vi "7p1_HW_Task1B_doanbs.vi"(6 "Units":string, 9 "Convert?":string, 10 "th, Theta":dbl, 11 "Trig Function":string) -> (2 "Calculated Value":dbl, 3 "Units Output":string)   [LabVIEW 2016]
uses:
  <vilib>/express/express arith-compare/Formula/XNode/ExpressFormulaBlockNode.xnode
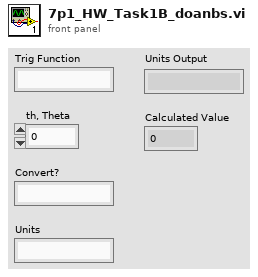
[diagram p1: front panel]
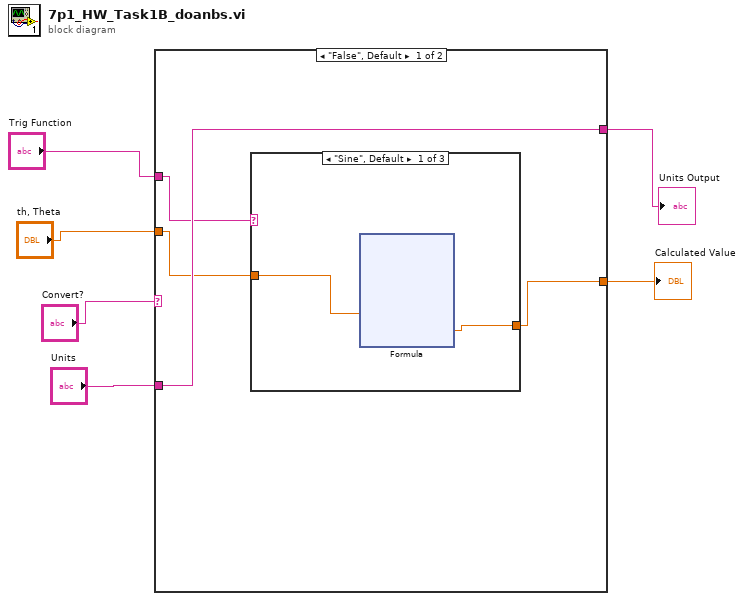
[diagram p0: block diagram]
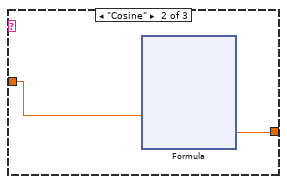
[diagram p2: hidden frame]
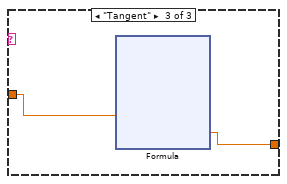
[diagram p3: hidden frame]
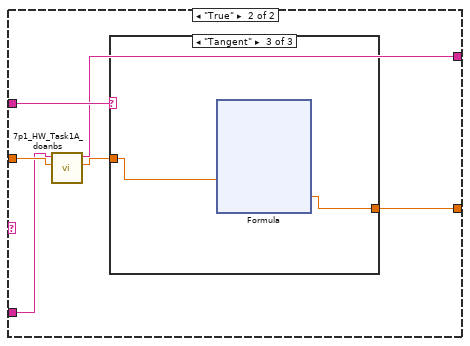
[diagram p4: hidden frame]
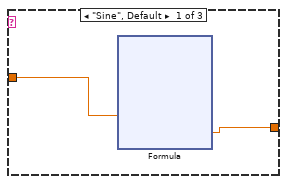
[diagram p5: hidden frame]
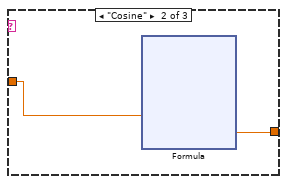
[diagram p6: hidden frame]
diagram:
  n1 = case shown="\"False\", Default" "Convert?" {
    tunnel: "Trig Function" -> [w7 w46]
    tunnel: "th, Theta" -> [w9 w45]
    tunnel: "Units" -> [w10 w44]
    tunnel: [w8 w41] -> w5
    tunnel: [w10 w42] -> w6
    frame "False", Default {
      n2 = case shown="\"Sine\", Default" w7 {
        tunnel: w9 -> [w12 w22 w32]
        tunnel: [w11 w21 w31] -> w8
        frame "Sine", Default {
          n3 = xnode "Formula"("th"=w12) -> ("Result"=w11:dbl)  [unwired: 1 in, 1 out]
        }
        frame "Cosine" {
          n4 = xnode "Formula"("th"=w22) -> ("Result"=w21:dbl)  [unwired: 1 in, 1 out]
        }
        frame "Tangent" {
          n5 = xnode "Formula"("th"=w32) -> ("Result"=w31:dbl)  [unwired: 1 in, 1 out]
        }
      }
    }
    frame "True" {
      n6 = call "7p1_HW_Task1A_doanbs.vi"("th, Theta in"=w45, "Units in"=w44) -> ("th, Theta out"=w43:dbl, "Units out"=w42:string)  [unwired: 8 in]
      n7 = case shown="\"Tangent\"" w46 {
        tunnel: w43 -> [w48 w58 w68]
        tunnel: [w47 w57 w67] -> w41
        frame "Sine", Default {
          n8 = xnode "Formula"("th"=w48) -> ("Result"=w47:dbl)  [unwired: 1 in, 1 out]
        }
        frame "Cosine" {
          n9 = xnode "Formula"("th"=w58) -> ("Result"=w57:dbl)  [unwired: 1 in, 1 out]
        }
        frame "Tangent" {
          n10 = xnode "Formula"("th"=w68) -> ("Result"=w67:dbl)  [unwired: 1 in, 1 out]
        }
      }
    }
  }
  "Units Output" <- w6
  "Calculated Value" <- w5
